vi "Retrieve L.vi"(10 "Matrix In":fxp<+,64,57>[](array[numeric])=[0.0, 0.0, 0.0, 0.0, 0.0, 0.0, 0.0, 0.0, 0.0]) -> (3 "L":fxp<+,64,57>[](array[numeric]) format="%.25g")   [LabVIEW 2014]
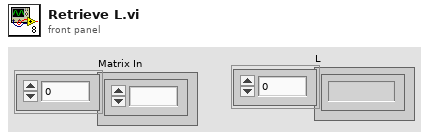
[diagram p1: front panel]
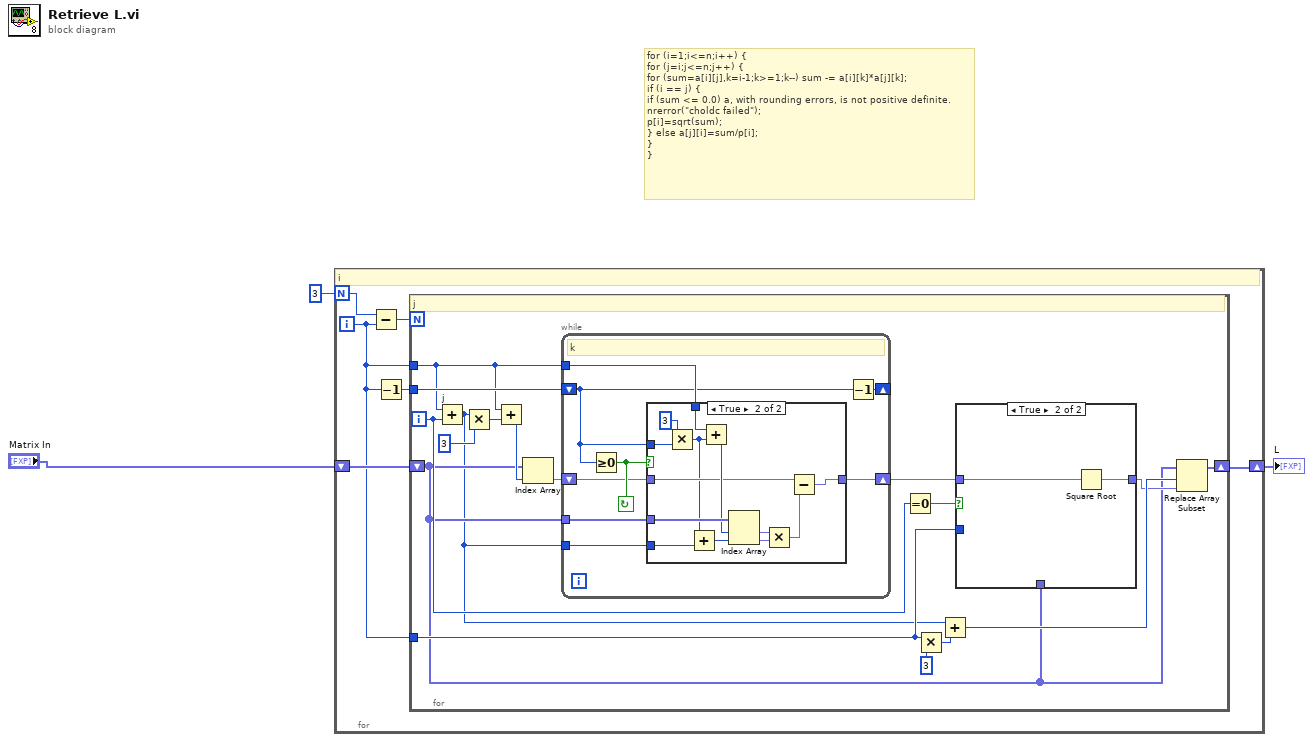
[diagram p0: block diagram]
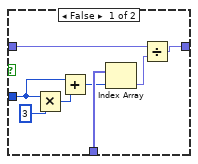
[diagram p2: hidden frame]
diagram:
  # "for (i=1;i<=n;i++) {\nfor (j=i;j<=n;j++) {\nfor (sum=a[i][j],k=i-1;k>=1;k--) sum -= a[i][k]*a[j][k];\nif (i == j) {\nif (sum <= 0.0) a, with rounding errors, is not positive definite.\nnrerror(\"choldc failed\");\np[i]=sqrt(sum);\n} else a[j][i]=sum/p[i];\n}\n}"
  n1 = for {
    N: 3 -> [w9]
    shift-right: [w4] -> w1
    shift-left: "Matrix In" -> [w6]
    i -> [w5]
    # "i"
    n2 = Subtract(x=w9, y=w5) -> (x-y=w8:i32)
    n3 = Decrement(x=w5) -> (x-1=w7:i32)
    n4 = for {
      N: w8 -> [_]
      tunnel: w7 -> [w26]
      tunnel: w5 -> [w22]
      tunnel: w5 -> [w12]
      shift-right: [w15] -> w4
      shift-left: w6 -> [w11]
      i -> [w18]
      # "j"
      n5 = Add "j"(x=w22, y=w18) -> (x+y=w10:i32)
      n6 = Multiply(x=w10, y=3) -> (x*y=w21:i32)
      n7 = Add(x=w22, y=w21) -> (x+y=w24:i32)
      n8 = Index Array(array=w11, index=w24) -> (element=w23:fxp<+,64,57>)
      n9 = while {
        shift-right: [w43] -> _
        shift-left: w26 -> [w39]
        shift-right: [w38] -> w19
        shift-left: w23 -> [w42]
        tunnel: w11 -> [w41]
        tunnel: w22 -> [w40]
        tunnel: w10 -> [w37]
        stop <- w44 continue-if-true
        # "k"
        n10 = Greater Or Equal To 0?(x=w39) -> (x >= 0?=w44:bool)
        n11 = case shown="True" w44 {
          tunnel: w42 -> [w45 w51]
          tunnel: w41 -> [_ w58]
          tunnel: w40 -> [_ w55]
          tunnel: w39 -> [_ w57]
          tunnel: [w45 w49] -> w38
          tunnel: w37 -> [_ w48]
          frame False {
          }
          frame True {
            n12 = Multiply(x=3 ("y"), y=w57) -> (x*y=w47:i32)
            n13 = Add(x=w47, y=w48) -> (x+y=w46:i32)
            n14 = Add(x=w55, y=w47) -> (x+y=w54:i32)
            n15 = Index Array(array=w58, index #1=w54, index #2=w46) -> (element #1=w53:fxp<+,64,57>, element #2=w52:fxp<+,64,57>)
            n16 = Multiply(x=w53, y=w52) -> (x*y=w50:fxp<+,64,57>)
            n17 = Subtract(x=w51, y=w50) -> (x-y=w49:fxp<+,64,57>)
          }
        }
        n18 = Decrement(x=w39) -> (x-1=w43:i32)
      }
      n19 = Equal To 0?(x=w18) -> (x = 0?=w20:bool)
      n20 = Multiply(x=w12, y=3 ("x")) -> (x*y=w16:i32)
      n21 = Add(x=w10, y=w16) -> (x+y=w14:i32)
      n22 = case shown="True" w20 {
        tunnel: w19 -> [w34 w36]
        tunnel: [w33 w35] -> w13
        tunnel: w12 -> [w30 _]
        tunnel: w11 -> [w29 _]
        frame False {
          n23 = Multiply(x=w30, y=3 ("x")) -> (x*y=w31:i32)
          n24 = Add(x=w30, y=w31) -> (x+y=w28:i32)
          n25 = Index Array(array=w29, index=w28) -> (element=w27:fxp<+,64,57>)
          n26 = Divide(x=w34, y=w27) -> (x/y=w33:fxp<+,64,57>)
        }
        frame True {
          n27 = Square Root(x=w36) -> (sqrt(x)=w35:fxp<+,64,57>)
        }
      }
      n28 = Replace Array Subset(array=w11, new element=w13, index=w14) -> (w15:fxp<+,64,57>[])
    }
  }
  "L" <- w1
